vi "re_LuaVIEW Kill Task_srv.vi"(7 "certificate":string, 11 "task identifier":string) -> (15 "error out":errorcluster)   [LabVIEW 2012]
doc: "Try to kill a task. This VI is reentrant because there is a small risk that the task VI is stuck on the C side which cause the VI abort method (which is used as a last resort) to hang without timing out (under LabVIEW 7.0 anyway). When the C code in question is called via Lua, this condition can be tested for and calling of the abort method is avoided. Unfortunately, it can also happen on the LabVIEW side, e.g. by calling some DLL function or VI-server method that does not return."
uses:
  clientsrv/typedefs/t_ClientSrv Access Levels.ctl
  typedefs/t_LuaVIEW Task List Methods.ctl
  typedefs/t_LuaVIEW Task State Methods.ctl
  typedefs/t_LuaVIEW Task Signals.ctl
  typedefs/t_LuaVIEW Task Modes.ctl
  typedefs/t_LuaVIEW CIN Spinlocked Actions.ctl
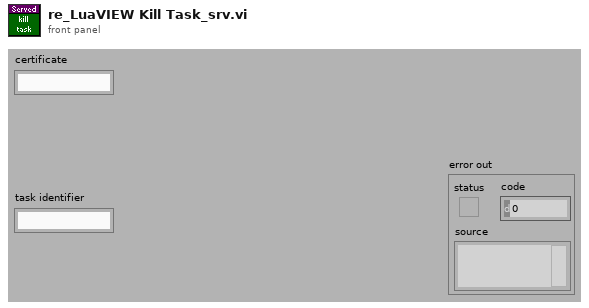
[diagram p1: front panel]
types:
  T1 = typedef "t_ClientSrv Access Levels.ctl" = enum16{"observer", "operator", "local"}
  T2 = typedef "t_LuaVIEW Task Signals.ctl" = enum32{"resume", "pause", "swap", "stop", "confirm"}
  T3 = typedef "t_LuaVIEW Task State Methods.ctl" = enum16{"cleanup", "set initial", "set mode", "set active mode", "set error", "get task info", "get script info", "set signal", "clear signal", "test handled", "test delegated", "test signal", "handle signal", "delegate signal", "allow signal", "disallow signal", "disallow all", "signals?", "delegated signals?", "protection++", "protection--", "protection=0", "message", "next message", "pop message", "message available?", "force stop", "set swap preps", "apply swap preps"}
  T4 = typedef "t_LuaVIEW Task List Methods.ctl" = enum16{"clear list", "add", "test", "remove", "get ref", "get task info", "get list", "get script info", "ongoing?", "resume", "pause", "stop", "confirm", "message"}
  T5 = typedef "t_LuaVIEW CIN Spinlocked Actions.ctl" = enum16{"totals", "taskcount", "open", "registerpublic", "registerexport", "revokeexports", "unregnextpublic", "usepublic", "pollexport", "close", "startyieldtest", "endyieldtest", "pollprintbuffer"}
  T6 = typedef "t_LuaVIEW Task Modes.ctl" = enum16{"initializing", "running", "executing", "paused", "error", "swapping"}
  T7 = typedef "t_LuaVIEW Task State Pane.ctl" = refnum<vi>
  T8 = typedef "LuaVIEW Task Info.ctl" = cluster{"main script":string, "identifier":string, "class":string, "description":string, "mode":T6, "handler":string, "LuaVIEW reference":T9, "scripts":i32, "hide":bool, "active":bool, "error msg":string, "defer":bool, "launch":enum16{"asynchronous", "manual", "synchronous"}, "main path valid":bool, "start time":dbl, "swap time":dbl, "task VI":refnum<vi>, "prefsys":enum32{"invalid execution system", "user interface", "standard", "instrument i/o", "data acquisition", "other 1", "other 2", "same as caller"}, "priority":enum32{"invalid priority", "background priority", "normal priority", "above normal priority", "high priority", "time critical priority", "subroutine"}, "signal flags":u32, "allow mask":u32, "handle mask":u32, "disallow manual":bool}
  T9 = typedef "t_LuaVIEW Reference.ctl" = refnum<k1>
  T10 = typedef "et_LuaVIEW CIN Results.ctl" = enum16{"OK", "error", "main", "call", "clonecall", "modulecall", "exportcall", "index", "yield"}
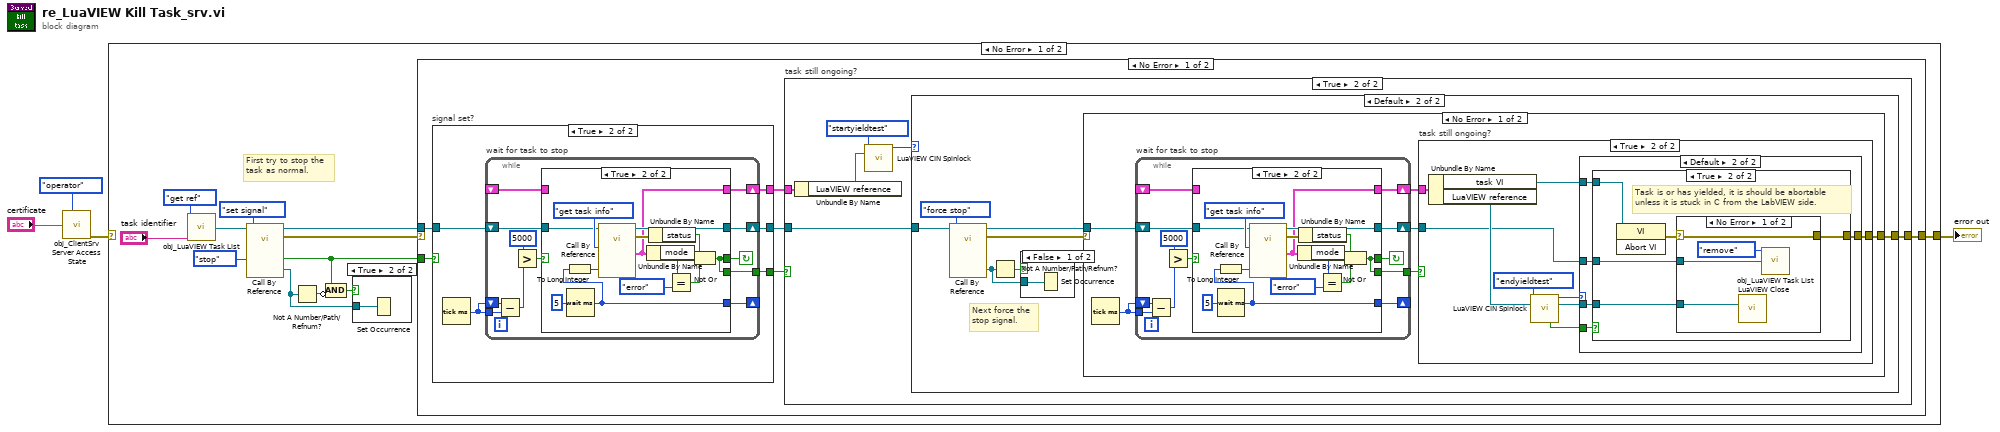
[diagram p0: block diagram]
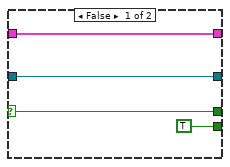
[diagram p4: hidden frame]
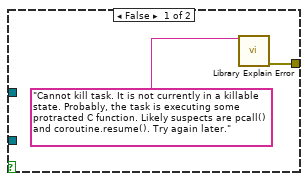
[diagram p7: hidden frame]
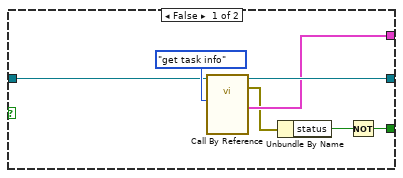
[diagram p11: hidden frame]
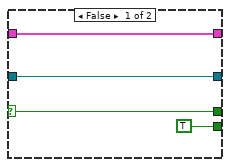
[diagram p12: hidden frame]
diagram:
  n1 = call "obj_ClientSrv Server Access State.vi"("access level"=t_ClientSrv_Access_Levels."operator", "certificate in"="certificate") -> ("error out"=w3:errorcluster)  [unwired: 11 in, 2 out]
  n2 = case shown="No Error" w3 {
    selector: w3 -> [_ w142]
    tunnel: [w15 w142] -> w4
    frame No Error {
      # "First try to stop the\ntask as normal."
      n3 = call "obj_LuaVIEW Task List.vi"("method"=t_LuaVIEW_Task_List_Methods."get ref", "task identifier"="task identifier") -> ("state object ref out"=w12:T7)  [unwired: 8 in, 5 out]
      n4 = call-by-ref "?"(reference=w12, "method"=t_LuaVIEW_Task_State_Methods."set signal", "signal"=t_LuaVIEW_Task_Signals."stop") -> (reference out=w6:T7, error out=w7:errorcluster, "set/available/pending"=w5:bool, "wakeup occurrence"=w8:refnum<k4>)  [unwired: 10 in, 3 out]
      n5 = Not A Number/Path/Refnum?(number/path/refnum=w8) -> (NaN/Path/Refnum?=w10:bool)
      n6 = Compound Arithmetic op=AND(w5, invert w10) -> (w9:bool)
      n7 = case shown="True" w9 {
        tunnel: w8 -> [_ w141]
        frame False {
        }
        frame True {
          n8 = Set Occurrence(w141) -> ()
        }
      }
      n9 = case shown="No Error" w7 {
        selector: w7 -> [_ w140]
        tunnel: [w22 w140] -> w15
        tunnel: w6 -> [w20 _]
        tunnel: w5 -> [w21 _]
        frame No Error {
          n10 = case "signal set?" shown="True" w21 {
            tunnel: w20 -> [w104 w110]
            tunnel: [w100 w109] -> w19
            tunnel: [w103 w108] -> w18
            tunnel: [w102 w106] -> w17
            frame False {
              n11 = call-by-ref "?"(reference=w104, "method"=t_LuaVIEW_Task_State_Methods."get task info") -> (reference out=w103:T7, error out=w101:errorcluster, "task info {get task info}"=w102:T8)  [unwired: 11 in, 4 out]
              n12 = Unbundle By Name(w101) -> ("status"=w99:bool)
              n13 = Not(x=w99) -> (.not. x?=w100:bool)
            }
            frame True {
              n14 = Tick Count (ms)() -> (millisecond timer value=w107:u32)
              n15 = while "wait for task to stop" {
                shift-right: [w121] -> w108
                shift-left: w110 -> [w122]
                tunnel: w107 -> [w119]
                tunnel: [w115] -> w109
                shift-right: [w114] -> w106
                shift-left: _ -> [w113]
                shift-right: [w111] -> _
                shift-left: w107 -> [w112]
                stop <- w120 continue-if-true
                n16 = Subtract(x=w112, y=w119) -> (x-y=w118:u32)
                n17 = Greater?(x=u32 5000, y=w118) -> (0:w116:bool)
                n18 = case shown="True" w116 {
                  selector: w116 -> [w126 _]
                  tunnel: w122 -> [w125 w133]
                  tunnel: [w125 w132] -> w121
                  tunnel: [w126 w131] -> w120
                  tunnel: [TRUE w131] -> w115
                  tunnel: [w123 w130] -> w114
                  tunnel: w113 -> [w123 _]
                  tunnel: [_ w127] -> w111
                  frame False {
                  }
                  frame True {
                    n19 = Wait (ms)(milliseconds to wait=u32 5) -> (millisecond timer value=w127:u32)
                    n20 = To Long Integer(number=w127) -> (32bit integer=w128:i32)
                    n21 = call-by-ref "?"(reference=w133, "method"=t_LuaVIEW_Task_State_Methods."get task info", "script index"=w128) -> (reference out=w132:T7, error out=w137:errorcluster, "task info {get task info}"=w130:T8)  [unwired: 10 in, 4 out]
                    n22 = Unbundle By Name(w130) -> ("mode"=w136:T6)
                    n23 = Unbundle By Name(w137) -> ("status"=w135:bool)
                    n24 = Equal?(x=w136, y=t_LuaVIEW_Task_Modes."error" ("mode")) -> (x = y?=w134:bool)
                    n25 = Not Or(1:w134, 2:w135) -> (0:w131:bool)
                  }
                }
              }
            }
          }
          n26 = case "task still ongoing?" shown="True" w19 {
            tunnel: [_ w28] -> w22
            tunnel: w18 -> [_ w27]
            tunnel: w17 -> [_ w26]
            frame False {
            }
            frame True {
              n27 = Unbundle By Name(w26) -> ("LuaVIEW reference"=w25:T9)
              n28 = call "LuaVIEW CIN Spinlock.vi"("action"=t_LuaVIEW_CIN_Spinlocked_Actions."startyieldtest", "LuaVIEW reference in"=w25) -> ("result"=w24:T10)  [unwired: 7 in, 6 out]
              n29 = case shown="Default" w24 {
                tunnel: [_ w30] -> w28
                tunnel: w27 -> [_ w29]
                frame "error" {
                }
                frame Default {
                  # "Next force the\nstop signal."
                  n30 = call-by-ref "?"(reference=w29, "method"=t_LuaVIEW_Task_State_Methods."force stop") -> (reference out=w32:T7, error out=w31:errorcluster, "wakeup occurrence"=w33:refnum<k4>)  [unwired: 11 in, 4 out]
                  n31 = Not A Number/Path/Refnum?(number/path/refnum=w33) -> (NaN/Path/Refnum?=w35:bool)
                  n32 = case shown="False" w35 {
                    tunnel: w33 -> [w98 _]
                    frame False {
                      n33 = Set Occurrence(w98) -> ()
                    }
                    frame True {
                    }
                  }
                  n34 = case shown="No Error" w31 {
                    selector: w31 -> [_ w97]
                    tunnel: w32 -> [w40 _]
                    tunnel: [w41 w97] -> w30
                    frame No Error {
                      n35 = Tick Count (ms)() -> (millisecond timer value=w37:u32)
                      n36 = while "wait for task to stop" {
                        shift-right: [w52] -> w36
                        shift-left: w40 -> [w53]
                        tunnel: w37 -> [w50]
                        tunnel: [w46] -> w38
                        shift-right: [w45] -> w39
                        shift-left: _ -> [w44]
                        shift-right: [w42] -> _
                        shift-left: w37 -> [w43]
                        stop <- w51 continue-if-true
                        n37 = Subtract(x=w43, y=w50) -> (x-y=w49:u32)
                        n38 = Greater?(x=u32 5000, y=w49) -> (0:w47:bool)
                        n39 = case shown="True" w47 {
                          selector: w47 -> [w57 _]
                          tunnel: w53 -> [w56 w64]
                          tunnel: [w56 w63] -> w52
                          tunnel: [w57 w62] -> w51
                          tunnel: [TRUE w62] -> w46
                          tunnel: [w54 w61] -> w45
                          tunnel: w44 -> [w54 _]
                          tunnel: [_ w58] -> w42
                          frame False {
                          }
                          frame True {
                            n40 = Wait (ms)(milliseconds to wait=u32 5) -> (millisecond timer value=w58:u32)
                            n41 = To Long Integer(number=w58) -> (32bit integer=w59:i32)
                            n42 = call-by-ref "?"(reference=w64, "method"=t_LuaVIEW_Task_State_Methods."get task info", "script index"=w59) -> (reference out=w63:T7, error out=w68:errorcluster, "task info {get task info}"=w61:T8)  [unwired: 10 in, 4 out]
                            n43 = Unbundle By Name(w61) -> ("mode"=w67:T6)
                            n44 = Unbundle By Name(w68) -> ("status"=w66:bool)
                            n45 = Equal?(x=w67, y=t_LuaVIEW_Task_Modes."error" ("mode")) -> (x = y?=w65:bool)
                            n46 = Not Or(1:w65, 2:w66) -> (0:w62:bool)
                          }
                        }
                      }
                      n47 = case "task still ongoing?" shown="True" w38 {
                        tunnel: w39 -> [_ w79]
                        tunnel: [_ w78] -> w41
                        tunnel: w36 -> [_ w71]
                        frame False {
                        }
                        frame True {
                          n48 = Unbundle By Name(w79) -> ("task VI"=w73:refnum<vi>, "LuaVIEW reference"=w76:T9)
                          n49 = call "LuaVIEW CIN Spinlock.vi"("action"=t_LuaVIEW_CIN_Spinlocked_Actions."endyieldtest", "LuaVIEW reference in"=w76) -> ("result"=w75:T10, "LuaVIEW reference out"=w72:T9, "boolean out"=w74:bool)  [unwired: 7 in, 4 out]
                          n50 = case shown="Default" w75 {
                            tunnel: [_ w84] -> w78
                            tunnel: w74 -> [_ w83]
                            tunnel: w73 -> [_ w82]
                            tunnel: w72 -> [_ w81]
                            tunnel: w71 -> [_ w80]
                            frame "error" {
                            }
                            frame Default {
                              n51 = case shown="True" w83 {
                                tunnel: [w85 w90] -> w84
                                tunnel: w82 -> [_ w89]
                                tunnel: w81 -> [_ w88]
                                tunnel: w80 -> [_ w87]
                                frame False {
                                n52 = call "Library Explain Error.vi"("explanation prefix (none)"="Cannot kill task. It is not currently in a killable state. Probably, the task is executing some protracted C function. Likely suspects are pcall() and coroutine.resume(). Try again later.") -> ("explained error"=w85:errorcluster)  [unwired: 14 in]
                                }
                                frame True {
                                # "Task is or has yielded, it is should be abortable\nunless it is stuck in C from the LabVIEW side."
                                n53 = invoke class="VI" method="Abort VI"(reference=w89) -> (error out=w91:errorcluster)  [unwired: 2 in, 2 out]
                                n54 = case shown="No Error" w91 {
                                selector: w91 -> [w95 w96]
                                tunnel: [w95 w96] -> w90
                                tunnel: w88 -> [w94 _]
                                tunnel: w87 -> [w93 _]
                                frame No Error {
                                n55 = call "LuaVIEW Close.vi"("LuaVIEW reference"=w94) -> ()  [unwired: 14 in, 1 out]
                                n56 = call "obj_LuaVIEW Task List.vi"("method"=t_LuaVIEW_Task_List_Methods."remove", "state object ref in"=w93) -> ()  [unwired: 8 in, 6 out]
                                }
                                frame Error {
                                }
                                }
                                }
                              }
                            }
                          }
                        }
                      }
                    }
                    frame Error {
                    }
                  }
                }
              }
            }
          }
        }
        frame Error {
        }
      }
    }
    frame Error {
    }
  }
  "error out" <- w4
